vi "Test Add and Undo All.vi"(8 "error in":errorcluster, 11 "Test Case In":refnum<class "Undo Redo Core.lvclass">) -> (0 "error out":errorcluster, 3 "Test Case Out":refnum<class "Undo Redo Core.lvclass">)   [LabVIEW 2020, in "Undo Redo Core.lvclass"]
doc: "Adds many states to the undo buffer and then performs an Undo on all of the added states."
uses:
  Undo Redo Core.lvclass
  <vilib>/Astemes/LUnit/Test Case.lvclass
panel:
  out "Have Changes":bool
  out "Undo Data":string[](array[string])
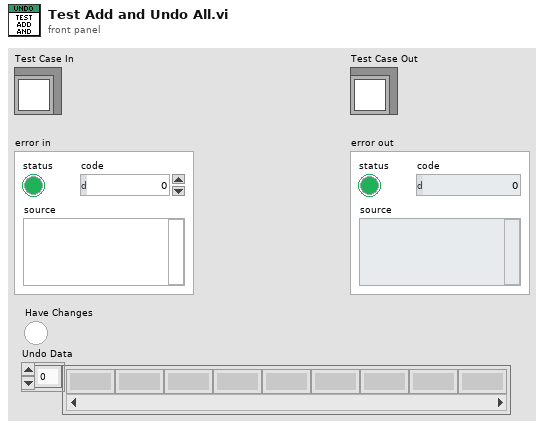
[diagram p1: front panel]
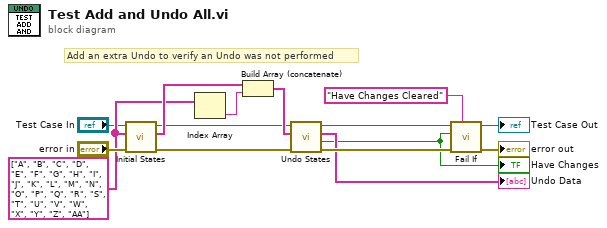
[diagram p0: block diagram]
diagram:
  w10 = string[] ["A", "B", "C", "D", "E", "F", "G", "H", "I", "J", "K", "L", "M", "N", "O", "P", "Q", "R", "S", "T", "U", "V", "W", "X", "Y", "Z", "AA"]
  # "Add an extra Undo to verify an Undo was not performed"
  n1 = call "Initial States.vi"("error in"="error in", "States"=w10, "Test Case In"="Test Case In") -> ("error out"=w14:errorcluster, "Expected Undo Stack"=w11:string[], "Test Case Out"=w6:refnum<class "Undo Redo Core.lvclass">)  [unwired: 5 in, 1 out]
  n2 = Index Array(array=w10) -> (element=w9:string)  [unwired: 1 in]
  n3 = Build Array (concatenate)(w11, w9) -> (w8:string[])
  n4 = call "Undo States.vi"("error in"=w14, "Expected Undo States"=w8, "Test Case In"=w6) -> ("error out"=w13:errorcluster, "Final Have Changes"=w3:bool, "Actual Undo States"=→"Undo Data":string[], "Test Case Out"=w5:refnum<class "Undo Redo Core.lvclass">)  [unwired: 5 in]
  "Have Changes" <- w3
  n5 = call <vilib>:"Fail If.vi"("Description"="Have Changes Cleared", "error in (no error)"=w13, "Fail?"=w3, "LUnit Test Case In"=w5) -> ("error out"=→"error out":errorcluster, "LUnit Test Case Out"=→"Test Case Out":refnum<class "Undo Redo Core.lvclass">)  [unwired: 6 in]
